vi "Delete Test File.vi"(11 "name or relative path":path=path "testdata") -> (0 "error out":errorcluster, 3 "deleted path":path)   [LabVIEW 2019]
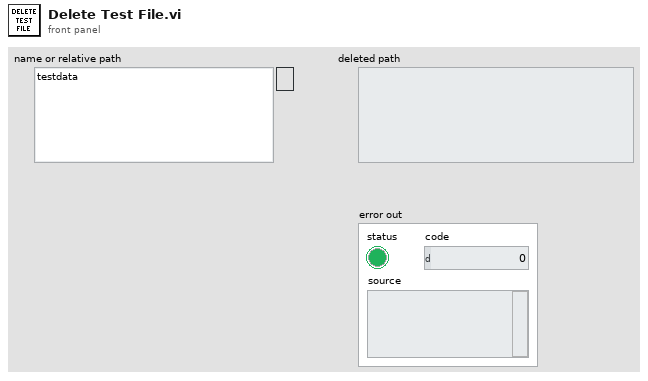
[diagram p1: front panel]
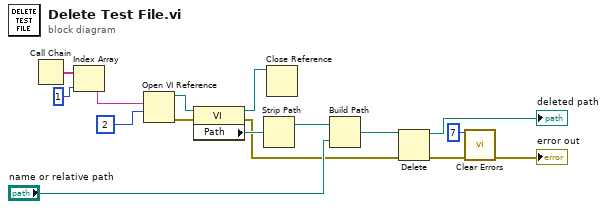
[diagram p0: block diagram]
diagram:
  n1 = Call Chain() -> (call chain=w9:string[])
  n2 = Index Array(array=w9, index=1 ("Index")) -> (element=w7:string)
  n3 = Open VI Reference(vi path=w7, options=2) -> (vi reference=w5:refnum<vi>, error out=w2:errorcluster)  [unwired: 4 in]
  n4 = property class="VI"(reference=w5, error in=w2) -> (reference out=w4:refnum<vi>, error out=w1:errorcluster, "Path"=w10:path)
  n5 = Strip Path(path=w10) -> (stripped path=w11:path)  [unwired: 1 out]
  n6 = Close Reference(reference=w4) -> ()  [unwired: 1 in, 1 out]
  n7 = Build Path(base path=w11, name or relative path="name or relative path") -> (appended path=w16:path)
  n8 = Delete(path (use dialog)=w16, error in=w1) -> (deleted path=→"deleted path":path, error out=w13:errorcluster)  [unwired: 3 in, 1 out]
  n9 = call <vilib>:"Clear Errors.vi"("error in (no error)"=w13, "specific error code to clear (0: all)"=7) -> ("error out"=→"error out":errorcluster)  [unwired: 4 in, 1 out]
